vi "getImageToArray.vi"(10 "New Image":T2, 11 "Session in":T1) -> (3 "imageGrayArray":u16[][](array[numeric]))   [LabVIEW 2021]
uses:
  <vilib>/vision/Image Controls.llb/IMAQ Image.ctl
  <vilib>/userdefined/High Color/IMAQdx.ctl
  <vilib>/vision/driver/IMAQdx.llb/IMAQdx Buffer Number Mode.ctl
  <vilib>/vision/driver/NI_Vision_Acquisition_Software.lvlib
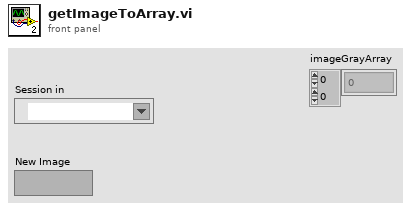
[diagram p1: front panel]
types:
  T1 = typedef "IMAQdx.ctl" = refnum<k21>
  T2 = typedef "IMAQ Image.ctl" = refnum<image>
  T3 = typedef "NI_Vision_Acquisition_Software.lvlib/IMAQdx Buffer Number Mode.ctl" = enum32{"Next", "Last", "Buffer Number", "Every", "Last New"}
  T4 = typedef "Image Type" = u32
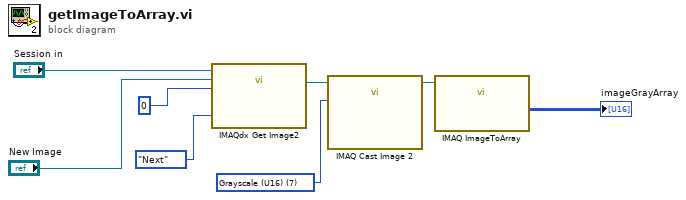
[diagram p0: block diagram]
diagram:
  w3 = T4 7 items=["Grayscale (U8)", "Grayscale (I16)", "Grayscale (SGL)", "Complex (CSG)", "RGB (U32)", "HSL (U32)", "RGB (U64)", "Grayscale (U16)"] ("Image Type")
  n1 = call <vilib>:"IMAQdx Get Image2.vi"("Buffer Number Mode (Next)"=IMAQdx_Buffer_Number_Mode."Next", "Buffer Number In"=u32 0, "Image In"="New Image", "Session In"="Session in") -> ("Image Out"=w5:T2)  [unwired: 4 in, 3 out]
  n2 = call "IMAQ Cast Image 2"("Image Src"=w5, "Image Type"=w3) -> ("Image Dst Out"=w8:T2)  [unwired: 12 in, 1 out]
  n3 = call "IMAQ ImageToArray"("Image"=w8) -> ("Image Pixels (U16)"=→"imageGrayArray":u16[][])  [unwired: 3 in, 4 out]
